vi "TestStand.DisplayExecutionCallback.vi"(4 "state variables in":T1={"DUTs.Name"=["All", "Station 1", "Station 2", "Station 3"], "Pages.Name"=[], "Pages.Ref"=[], "TS.UI"={"References"={"Event Callback"=refnum, "Quit Application Event"=refnum, "Events"=refnum, "Top level VI"=refnum, "TestStand Engine"=refnum, "Start Application Event"=refnum, "Stop Application Event"=refnum}, "Managers"={"Application Manager"=refnum, "SequenceFileView Manager"=refnum, "ExecutionView Manager"=refnum}, "Controls"={"Execution View"=refnum, "Run Button"=refnum, "Open Button"=refnum}}, "TS.Running"=FALSE, "TS.Abort"=FALSE, "NIVS.GatewayIPAddress"="", "NIVS.WorkspaceManager"=refnum, "NIVS.Open"=FALSE, "NIVS.Deployed"=FALSE, "NIVS.SystemStateRefs"={"CustDatRef"=refnum, "EvtRef"=refnum, "Target State User Event"=refnum}, "NIVS.Events"={"SystemChangeEvent"=refnum, "WorkspaceEvent"=refnum, "WaveformEvent"=refnum}, "UI.Tree"=refnum, "UI.Path"=refnum, "UI.Stop"=refnum, "UI.Tab"=refnum, "VI.Ref"=refnum}, 5 "Event data":cluster{"exec":refnum<k7>, "reason":i32}, 6 "CtlRef":refnum<k7>, 7 "Event common data":cluster{"Source":i32, "Type":u32, "Time":u32}) -> ()   [LabVIEW 2015, in "Main.GUI.lvlib"]
uses:
  Main.GUI.lvlib
  Types/Multihead.StateVariables.ctl
  Types/TestStandGUI.Refs.ctl
  <vilib>/NI Veristand/Execution/Workspace/WorkspaceAPI.ctl
  NationalInstruments.VeriStand.ClientAPI
  <vilib>/NI Veristand/Execution/Workspace/SystemStateEventRef.ctl
  <vilib>/NI Veristand/Execution/Workspace/Target State Info.ctl
  <vilib>/NI Veristand/Execution/Workspace/Target State.ctl
  Execution GUI/Types/Execute.UserEventRefs.ctl
  <vilib>/NI Veristand/Execution/Workspace/SystemStateRegEventRef.ctl
  <vilib>/NI Veristand/Execution/WaveformStreaming/Waveform Data Watcher Event Data (DBL).ctl
  <vilib>/NI Veristand/Execution/WaveformStreaming/WaveformStreamSpecification.ctl
  <vilib>/NI Veristand/Execution/Workspace/NI_VS Workspace ExecutionAPI.lvlib
  Execution GUI/Station.Execution.lvlib
  <vilib>/NI Veristand/Execution/WaveformStreaming/NI_VS Waveform Streaming Interface.lvlib
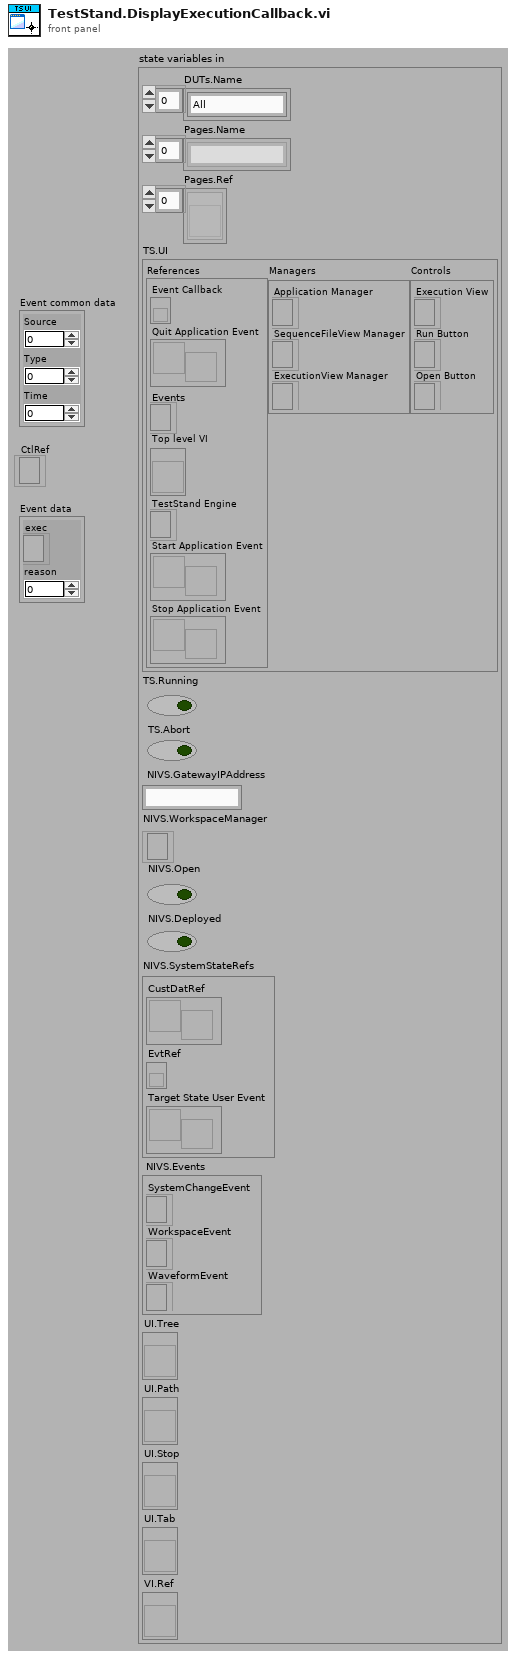
[diagram p1: front panel]
types:
  T1 = typedef "Main.GUI.lvlib/Multihead.StateVariables.ctl" = cluster{"DUTs.Name":string[], "Pages.Name":string[], "Pages.Ref":refnum<vi>[], "TS.UI":T2, "TS.Running":bool, "TS.Abort":bool, "NIVS.GatewayIPAddress":string, "NIVS.WorkspaceManager":T3, "NIVS.Open":bool, "NIVS.Deployed":bool, "NIVS.SystemStateRefs":T4, "NIVS.Events":T5, "UI.Tree":refnum<vi>, "UI.Path":refnum<vi>, "UI.Stop":refnum<vi>, "UI.Tab":refnum<vi>, "VI.Ref":refnum<vi>}
  T2 = typedef "Main.GUI.lvlib/TestStandGUI.Refs.ctl" = cluster{"References":cluster{"Event Callback":refnum<k27>, "Quit Application Event":refnum<user-event>, "Events":refnum<event-registration>, "Top level VI":refnum<vi>, "TestStand Engine":refnum<k7>, "Start Application Event":refnum<user-event>, "Stop Application Event":refnum<user-event>}, "Managers":cluster{"Application Manager":refnum<k7>, "SequenceFileView Manager":refnum<k7>, "ExecutionView Manager":refnum<k7>}, "Controls":cluster{"Execution View":refnum<k7>, "Run Button":refnum<k7>, "Open Button":refnum<k7>}}
  T3 = typedef "NI_VS Workspace ExecutionAPI.lvlib/WorkspaceAPI.ctl" = refnum<k24>
  T4 = typedef "NI_VS Workspace ExecutionAPI.lvlib/SystemStateEventRef.ctl" = cluster{"CustDatRef":refnum<user-event>, "EvtRef":refnum<k27>, "Target State User Event":refnum<user-event>}
  T5 = typedef "Station.Execution.lvlib/Execute.UserEventRefs.ctl" = cluster{"SystemChangeEvent":T6, "WorkspaceEvent":refnum<event-registration>, "WaveformEvent":refnum<event-registration>}
  T6 = typedef "NI_VS Workspace ExecutionAPI.lvlib/SystemStateRegEventRef.ctl" = refnum<event-registration>
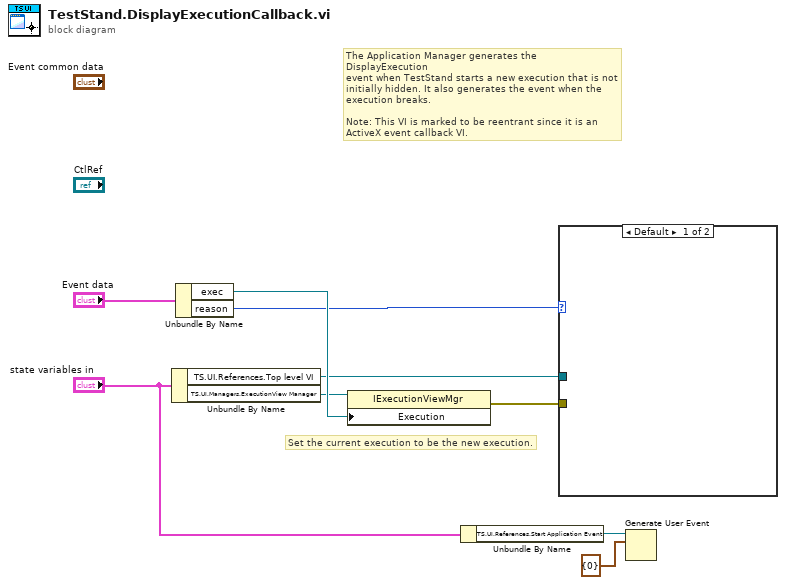
[diagram p0: block diagram]
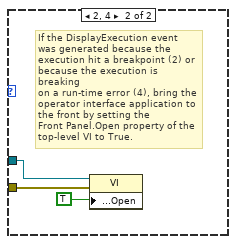
[diagram p2: hidden frame]
diagram:
  # "The Application Manager generates the DisplayExecution\nevent when TestStand starts a new execution that is not\ninitially hidden. It also generates the event when the\nexecution breaks.\n\nNote: This VI is marked to be reentrant since it is an\nActiveX event callback VI."
  # "Set the current execution to be the new execution."
  n1 = Unbundle By Name("state variables in") -> ("TS.UI.References.Top level VI"=w5:refnum<vi>, "TS.UI.Managers.ExecutionView Manager"=w6:refnum<k7>)
  n2 = Unbundle By Name("Event data") -> ("exec"=w9:refnum<k7>, "reason"=w7:i32)
  n3 = property class="IExecutionViewMgr"(reference=w6, "Execution"=w9) -> (error out=w4:errorcluster)  [unwired: 1 in, 1 out]
  n4 = Unbundle By Name("state variables in") -> ("TS.UI.References.Start Application Event"=w2:refnum<user-event>)
  n5 = case shown="Default" w7 {
    tunnel: w4 -> [_ w12]
    tunnel: w5 -> [_ w10]
    frame Default {
    }
    frame 2, 4 {
      # "If the DisplayExecution event\nwas generated because the\nexecution hit a breakpoint (2) or\nbecause the execution is breaking\non a run-time error (4), bring the\noperator interface application to\nthe front by setting the\nFront Panel.Open property of the\ntop-level VI to True."
      n6 = property class="VI"(reference=w10, error in=w12, "Front Panel Window:Open"=TRUE) -> ()  [unwired: 2 out]
    }
  }
  n7 = Generate User Event(user event=w2, event data cluster=cluster{i32} {0}) -> ()  [unwired: 2 in, 2 out]
